vi "Move Position.vi"(8 "error in (no error)":errorcluster caption="Error In", 10 "Position":T1, 11 "Array Ref":refnum<vi>) -> (0 "error out":errorcluster caption="Error Out", 1 "OK?":bool, 3 "Index":cluster{i32, u32, "Value":dbl})   [LabVIEW 2020]
uses:
  <vilib>/Utility/miscctls.llb/LVPositionTypeDef.ctl
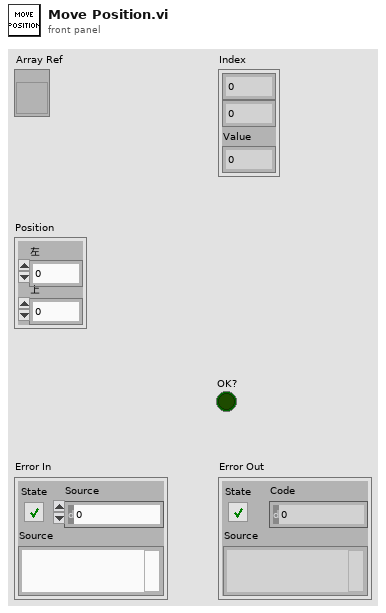
[diagram p1: front panel]
types:
  T1 = typedef "LVPositionTypeDef.ctl" = cluster{"Left":i32, "Top":i32}
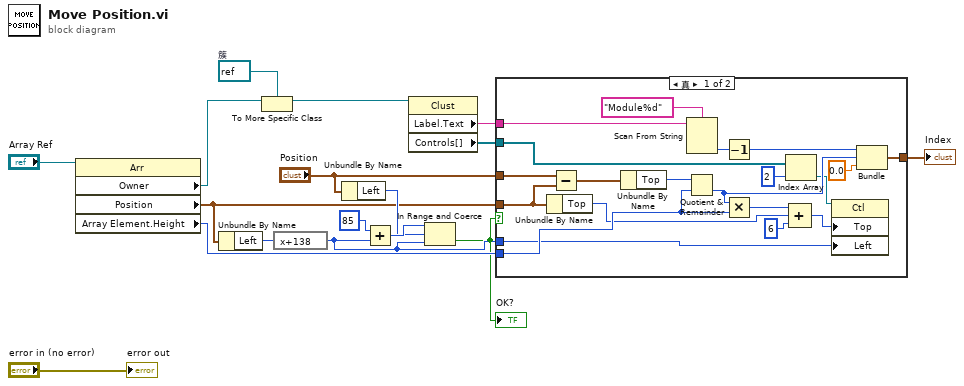
[diagram p0: block diagram]
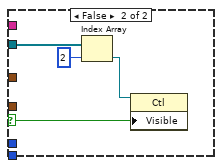
[diagram p2: hidden frame]
diagram:
  w5 = refnum<vi> refnum  # 簇
  n1 = property class="Arr"(reference="Array Ref") -> ("Owner"=w1:refnum<vi>, "Position"=w9:T1, "Array Element.Height"=w17:u32)  [unwired: 1 in, 2 out]
  n2 = Unbundle By Name(w9) -> ("Left"=w8:i32)
  n3 = To More Specific Class(target class=w5, reference=w1) -> (specific class reference=w4:refnum<vi>)  [unwired: 1 in, 1 out]
  n4 = expression code="x+138"(w8) -> (w7:i32)
  n5 = Unbundle By Name("Position") -> ("Left"=w11:i32)
  n6 = Add(x=85 ("Top"), y=w7) -> (x+y=w12:i32)
  n7 = property class="Clust"(reference=w4) -> ("Label.Text"=w2:string, "Controls[]"=w3:refnum<vi>[])  [unwired: 1 in, 2 out]
  n8 = In Range and Coerce(upper limit=w12, x=w11, lower limit=w7) -> (In Range?=w6:bool)  [unwired: 1 out]
  "OK?" <- w6
  n9 = case shown="真" w6 {
    selector: w6 -> [_ w39]
    tunnel: w17 -> [w35 _]
    tunnel: w9 -> [w32 _]
    tunnel: [w26 _] -> w15
    tunnel: "Position" -> [w25 _]
    tunnel: w7 -> [w24 _]
    tunnel: w3 -> [w18 w38]
    tunnel: w2 -> [w19 _]
    frame True {
      n10 = Unbundle By Name(w32) -> ("Top"=w31:i32)
      n11 = Subtract(x=w25, y=w32) -> (x-y=w37:T1)
      n12 = Unbundle By Name(w37) -> ("Top"=w36:i32)
      n13 = Scan From String(format string="Module%d" ("格式字符串"), input string=w19) -> (output 1=w27:i32)  [unwired: 3 in, 3 out]
      n14 = Quotient & Remainder(x=w36, y=w35) -> (floor(x/y)=w29:u32)  [unwired: 1 out]
      n15 = Decrement(x=w27) -> (x-1=w22:i32)
      n16 = Multiply(x=w29, y=w35) -> (x*y=w34:u32)
      n17 = Index Array(array=w18, index=2 ("索引")) -> (element=w20:refnum<vi>)
      n18 = Compound Arithmetic op=ADD(w34, w31, u32 6 ("y")) -> (w30:u32)
      n19 = property class="Ctl"(reference=w20, "Top"=w30, "Left"=w24) -> ()  [unwired: 1 in, 2 out]
      n20 = Bundle(w22, w29, 0.0) -> (w26:cluster{i32, u32, dbl})  [unwired: 1 in]
    }
    frame False {
      n21 = Index Array(array=w38, index=2 ("索引")) -> (element=w40:refnum<vi>)
      n22 = property class="Ctl"(reference=w40, "Visible"=w39) -> ()  [unwired: 1 in, 2 out]
    }
  }
  "Index" <- w15
  "error out" <- "error in (no error)"
